vi "Variant To Data_Binary.vi"(8 "error in (no error)":errorcluster, 11 "Variant":variant) -> (0 "error out":errorcluster, 2 "OK?":bool, 3 "Data Cluster":cluster{"Data":bool[]}[](array[cluster]))   [LabVIEW 2020, in "SECS Communication.lvlib" / "SECS-II Class.lvclass"]
uses:
  SECS-II Class.lvclass
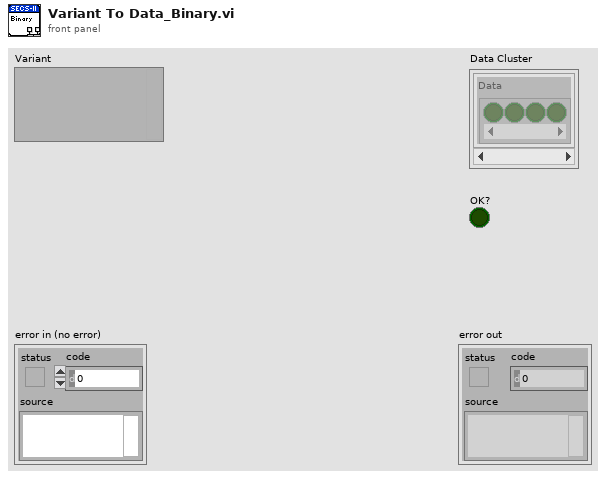
[diagram p1: front panel]
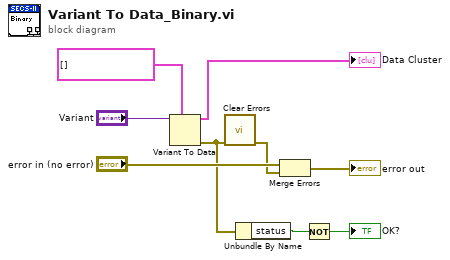
[diagram p0: block diagram]
diagram:
  n1 = Variant To Data(type=cluster{"Data":bool[]}[] [] ("Data Cluster"), Variant="Variant") -> (data=→"Data Cluster":cluster{"Data":bool[]}[], error out=w3:errorcluster)  [unwired: 1 in]
  n2 = call <vilib>:"Clear Errors.vi"("error in (no error)"=w3) -> ("error out"=w4:errorcluster)  [unwired: 5 in, 1 out]
  n3 = Unbundle By Name(w3) -> ("status"=w2:bool)
  n4 = Merge Errors("error in (no error)", w4) -> (→"error out":errorcluster)
  n5 = Not(x=w2) -> (.not. x?=→"OK?":bool)
